vi "ENPIDv2.vi"(0 "Gains":T6, 1 "Non-linear gain":T1, 2 "D-Part variable":T4, 3 "Velocity estimate dy/dt":T3, 4 "Anti reset windup":bool, 5 "I-Part error band":dbl=inf, 6 "Output range":T5, 7 "Reset?":bool, 8 "y":dbl, 9 "r":dbl, 11 "dy/dt":dbl, 13 "dt (s)":dbl) -> (15 "u":dbl, 18 "u":cluster{"up":dbl, "ui":dbl, "ud":dbl})   [LabVIEW 2015]
uses:
  Gains.ctl
  OutputRange.ctl
  DPartVariable.ctl
  VelocityEstimate.ctl
  NonLinearGainParams.ctl
  NonLinearGain.ctl
panel:
  # "Params"
  # "Input"
  # "Output"
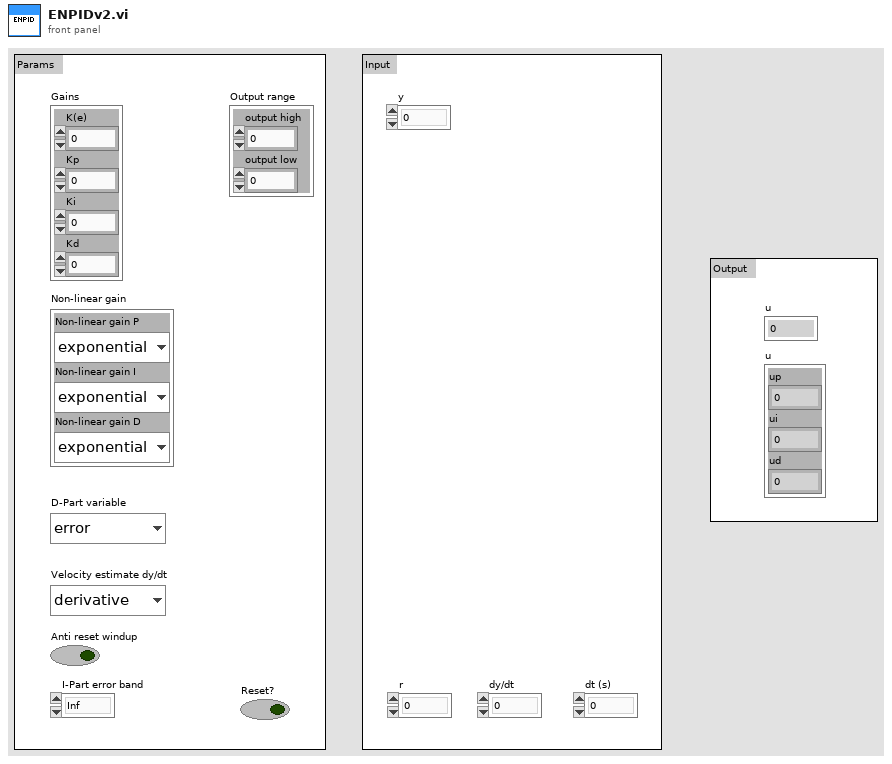
[diagram p1: front panel]
types:
  T1 = typedef "NonLinearGainParams.ctl" = cluster{"Non-linear gain P":T2, "Non-linear gain I":T2, "Non-linear gain D":T2}
  T2 = typedef "NonLinearGain.ctl" = enum16{"exponential", "quadratic", "off"}
  T3 = typedef "VelocityEstimate.ctl" = enum16{"derivative", "external"}
  T4 = typedef "DPartVariable.ctl" = enum16{"error", "process variable"}
  T5 = typedef "OutputRange.ctl" = cluster{"output high":dbl, "output low":dbl}
  T6 = typedef "Gains.ctl" = cluster{"K(e)":dbl, "Kp":dbl, "Ki":dbl, "Kd":dbl}
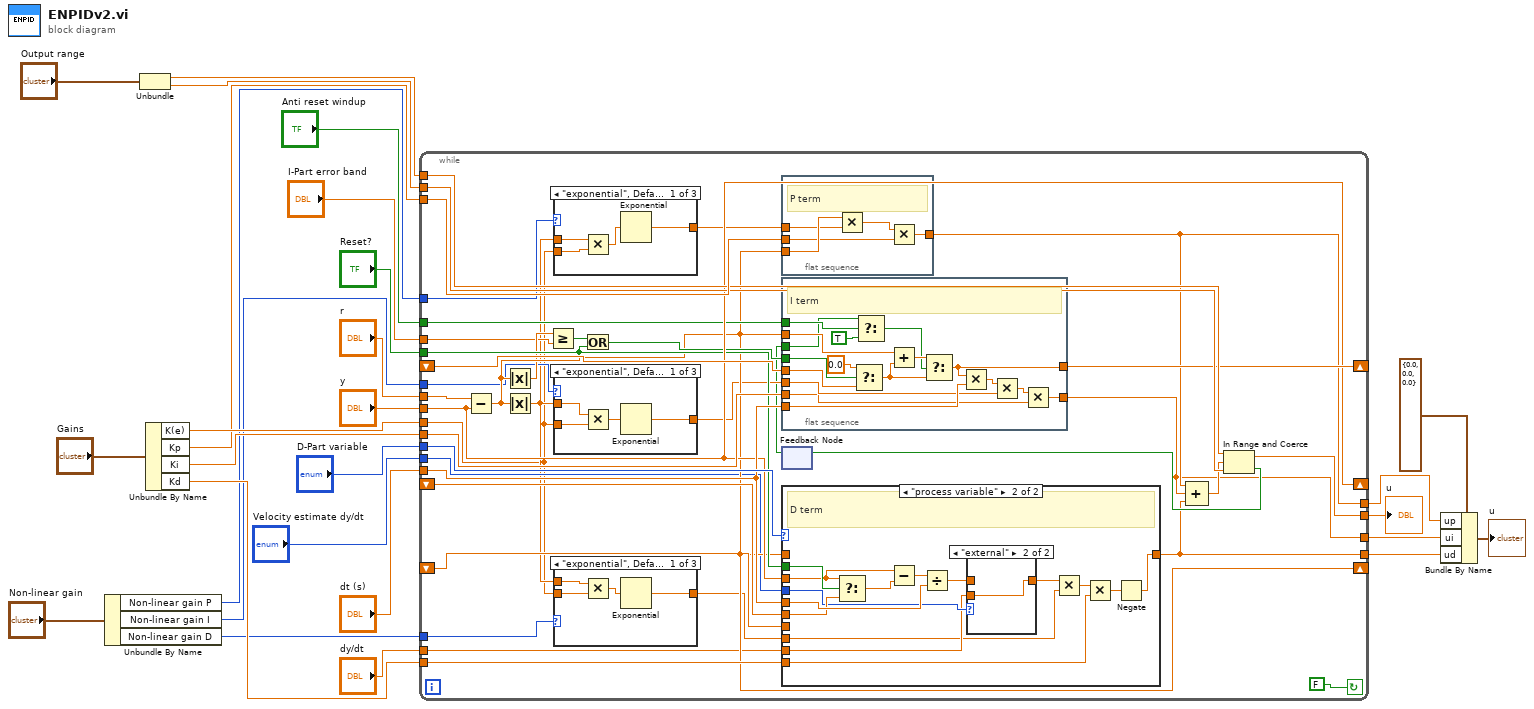
[diagram p0: block diagram]
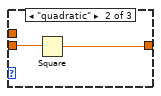
[diagram p2: hidden frame]
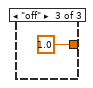
[diagram p3: hidden frame]
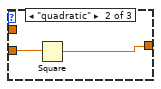
[diagram p4: hidden frame]
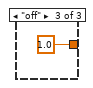
[diagram p5: hidden frame]
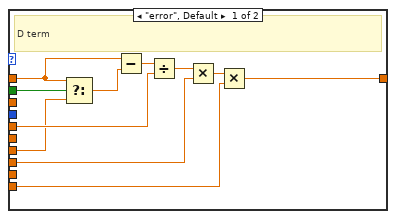
[diagram p6: hidden frame]
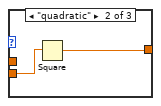
[diagram p8: hidden frame]
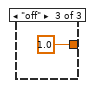
[diagram p9: hidden frame]
diagram:
  n1 = Unbundle By Name("Non-linear gain") -> ("Non-linear gain P"=w1:T2, "Non-linear gain I"=w3:T2, "Non-linear gain D"=w2:T2)
  n2 = Unbundle("Output range") -> ("output high"=w19:dbl, "output low"=w20:dbl)
  n3 = Unbundle By Name("Gains") -> ("K(e)"=w26:dbl, "Kp"=w22:dbl, "Ki"=w16:dbl, "Kd"=w14:dbl)
  n4 = while {
    tunnel: w26 -> [w34]
    tunnel: "r" -> [w65]
    tunnel: "y" -> [w52]
    tunnel: w22 -> [w64]
    shift-right: [w41] -> _
    shift-left: _ -> [w49]
    tunnel: [w62] -> w21
    tunnel: w20 -> [w61]
    tunnel: w19 -> [w60]
    tunnel: "Reset?" -> [w44]
    tunnel: "dt (s)" -> [w54]
    tunnel: w16 -> [w55]
    shift-right: [w58] -> _
    shift-left: _ -> [w57]
    tunnel: "D-Part variable" -> [w56]
    tunnel: w14 -> [w53]
    shift-right: [w52] -> _
    shift-left: _ -> [w51]
    tunnel: [w48] -> w11
    tunnel: [w47] -> w10
    tunnel: [w46] -> w9
    tunnel: "Anti reset windup" -> [w45]
    tunnel: "I-Part error band" -> [w39]
    tunnel: "dy/dt" -> [w38]
    tunnel: "Velocity estimate dy/dt" -> [w37]
    tunnel: w3 -> [w36]
    tunnel: w2 -> [w33]
    tunnel: w1 -> [w32]
    stop <- FALSE continue-if-true
    n5 = Subtract(x=w65, y=w52) -> (x-y=w41:dbl)
    n6 = Absolute Value(x=w41) -> (abs(x)=w40:dbl)
    n7 = Absolute Value(x=w41) -> (abs(x)=w35:dbl)
    n8 = Greater Or Equal?(x=w40, y=w39) -> (x >= y?=w42:bool)
    n9 = case shown="\"exponential\", Default" w32 {
      tunnel: w34 -> [w131 w135 _]
      tunnel: [w133 w134 1.0] -> w31
      tunnel: w35 -> [w130 _ _]
      frame "exponential", Default {
        n10 = Multiply(x=w130, y=w131) -> (x*y=w132:dbl)
        n11 = Exponential(1:w132) -> (0:w133:dbl)
      }
      frame "quadratic" {
        n12 = Square(x=w135) -> (x^2=w134:dbl)
      }
      frame "off" {
      }
    }
    n13 = case shown="\"exponential\", Default" w36 {
      tunnel: w34 -> [w74 w78 _]
      tunnel: [w76 w77 1.0] -> w29
      tunnel: w35 -> [w73 _ _]
      frame "exponential", Default {
        n14 = Multiply(x=w73, y=w74) -> (x*y=w75:dbl)
        n15 = Exponential(1:w75) -> (0:w76:dbl)
      }
      frame "quadratic" {
        n16 = Square(x=w78) -> (x^2=w77:dbl)
      }
      frame "off" {
      }
    }
    n17 = case shown="\"exponential\", Default" w33 {
      tunnel: w34 -> [w67 w71 _]
      tunnel: [w69 w70 1.0] -> w30
      tunnel: w35 -> [w66 _ _]
      frame "exponential", Default {
        n18 = Multiply(x=w66, y=w67) -> (x*y=w68:dbl)
        n19 = Exponential(1:w68) -> (0:w69:dbl)
      }
      frame "quadratic" {
        n20 = Square(x=w71) -> (x^2=w70:dbl)
      }
      frame "off" {
      }
    }
    n21 = Or(x=w42, y=w44) -> (x .or. y?=w43:bool)
    n22 = flat-sequence {
      tunnel: w41 -> [w129]
      tunnel: w31 -> [w125]
      tunnel: w64 -> [w127]
      tunnel: [w126] -> w48
      frame #0 {
        # "P term"
        n23 = Multiply(x=w129, y=w125) -> (x*y=w128:dbl)
        n24 = Multiply(x=w128, y=w127) -> (x*y=w126:dbl)
      }
    }
    n25 = flat-sequence {
      tunnel: w41 -> [w124]
      tunnel: w43 -> [w122]
      tunnel: w54 -> [w119]
      tunnel: w29 -> [w117]
      tunnel: w55 -> [w115]
      tunnel: [w114] -> w47
      tunnel: [w113] -> w58
      tunnel: w57 -> [w112]
      tunnel: w28 -> [w109]
      tunnel: w45 -> [w111]
      frame #0 {
        # "I term"
        n26 = Select(t=0.0, s=w122, f=w112) -> (s? t:f=w120:dbl)
        n27 = Select(t=w109, s=w111, f=TRUE) -> (s? t:f=w108:bool)
        n28 = Add(x=w124, y=w120) -> (x+y=w121:dbl)
        n29 = Select(t=w121, s=w108, f=w120) -> (s? t:f=w113:dbl)
        n30 = Multiply(x=w113, y=w119) -> (x*y=w118:dbl)
        n31 = Multiply(x=w118, y=w117) -> (x*y=w116:dbl)
        n32 = Multiply(x=w116, y=w115) -> (x*y=w114:dbl)
      }
    }
    n33 = feedback #1() -> (w28:bool)  [unwired: 1 in]
    n34 = case shown="\"process variable\"" w56 {
      tunnel: w41 -> [w82 _]
      tunnel: w49 -> [w83 _]
      tunnel: w54 -> [w89 w103]
      tunnel: w30 -> [w80 w91]
      tunnel: w53 -> [w86 w104]
      tunnel: [w85 w101] -> w46
      tunnel: w52 -> [_ w96]
      tunnel: w51 -> [_ w98]
      tunnel: w44 -> [w84 w99]
      tunnel: w38 -> [_ w94]
      tunnel: w37 -> [_ w95]
      frame "error", Default {
        # "D term"
        n35 = Select(t=w82, s=w84, f=w83) -> (s? t:f=w81:dbl)
        n36 = Subtract(x=w82, y=w81) -> (x-y=w90:dbl)
        n37 = Divide(x=w90, y=w89) -> (x/y=w88:dbl)
        n38 = Multiply(x=w88, y=w80) -> (x*y=w87:dbl)
        n39 = Multiply(x=w87, y=w86) -> (x*y=w85:dbl)
      }
      frame "process variable" {
        # "D term"
        n40 = Select(t=w96, s=w99, f=w98) -> (s? t:f=w97:dbl)
        n41 = Subtract(x=w96, y=w97) -> (x-y=w102:dbl)
        n42 = Divide(x=w102, y=w103) -> (x/y=w93:dbl)
        n43 = case shown="\"external\"" w95 {
          tunnel: w94 -> [_ w107]
          tunnel: [w106 w107] -> w92
          tunnel: w93 -> [w106 _]
          frame "derivative", Default {
          }
          frame "external" {
          }
        }
        n44 = Multiply(x=w92, y=w91) -> (x*y=w105:dbl)
        n45 = Multiply(x=w105, y=w104) -> (x*y=w100:dbl)
        n46 = Negate(x=w100) -> (-x=w101:dbl)
      }
    }
    n47 = Compound Arithmetic op=ADD(w48, w47, w46) -> (w59:dbl)
    n48 = In Range and Coerce(upper limit=w60, x=w59, lower limit=w61) -> (coerced(x)=w62:dbl, In Range?=w50:bool)
    n49 = feedback-in #1(w50) -> ()
  }
  "u" <- w21
  n50 = Bundle By Name(cluster=cluster{"up":dbl, "ui":dbl, "ud":dbl} {"up"=0.0, "ui"=0.0, "ud"=0.0}, "up"=w11, "ui"=w10, "ud"=w9) -> (→"u":cluster{"up":dbl, "ui":dbl, "ud":dbl})
